vi "Returns_to_tabs.vi"(1 "Input string":string) -> (0 "Output string":string)   [LabVIEW 2010]
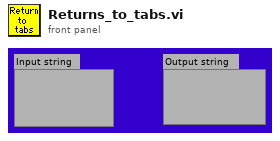
[diagram p1: front panel]
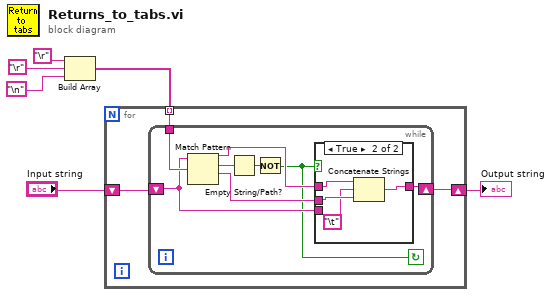
[diagram p0: block diagram]
diagram:
  n1 = Build Array("\r", "\r", "\n") -> (w4:string[])
  n2 = for {
    tunnel: w4 -> [w9] mode=indexing
    shift-right: [w7] -> w2
    shift-left: "Input string" -> [w8]
    n3 = while {
      shift-left: w8 -> [w13]
      shift-right: [w14] -> w7
      tunnel: w9 -> [w17]
      stop <- w10 continue-if-true
      n4 = Match Pattern(string=w13, regular expression=w17) -> (before substring=w12:string, match substring=w16:string, after substring=w11:string)  [unwired: 2 out]
      n5 = Empty String/Path?(string/path=w16) -> (empty?=w15:bool)
      n6 = Not(x=w15) -> (.not. x?=w10:bool)
      n7 = case shown="True" w10 {
        tunnel: [w18 w21] -> w14
        tunnel: w13 -> [w18 _]
        tunnel: w12 -> [_ w22]
        tunnel: w11 -> [_ w20]
        frame False {
        }
        frame True {
          n8 = Concatenate Strings(w22, "\t", w20) -> (w21:string)
        }
      }
    }
  }
  "Output string" <- w2
